vi "configureAnalogOutput.vi"(8 "error in (no error)":errorcluster, 9 "AnalogOutput":refnum<class "AnalogOutput.lvclass">, 10 "deviceName":string, 11 "AtomChipHWC in":refnum<class "AtomChipHWC.lvclass">) -> (0 "error out":errorcluster, 3 "AtomChipHWC out":refnum<class "AtomChipHWC.lvclass">)   [LabVIEW 2009, in "Hardware.lvlib" / "HWControllers.lvlib" / "AtomChipHWC.lvclass"]
doc: "Configure the analog channels of a device"
uses:
  AtomChipHWC.lvclass
  Channels/VoltOutput/AnalogOutput.lvclass
  AtomChipHWC.lvclass/AtomChipHWC.ctl
  HWController.lvclass
  Tools/Filing/FileNeologist/FileNeologist.lvclass
  Tools/Filing.lvlib
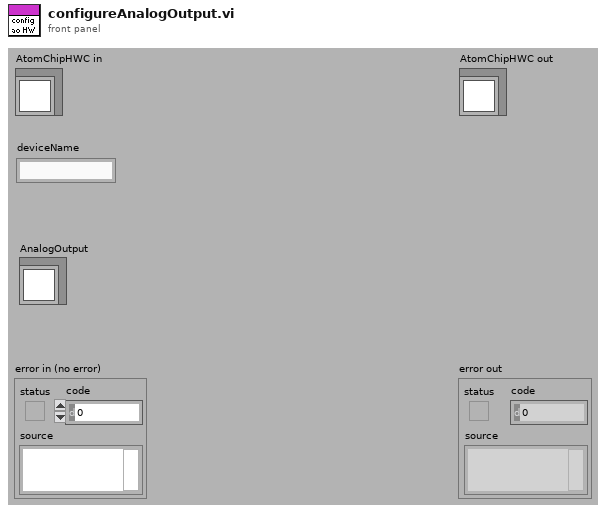
[diagram p1: front panel]
types:
  T1 = cluster{string, "Physical Channels":string, "Ranges":dbl[]}
  T2 = cluster{"Clock source":string, "Clock rate":dbl, "Start trigger line":string, "Sample Rate":dbl, "Sample No.":dbl}
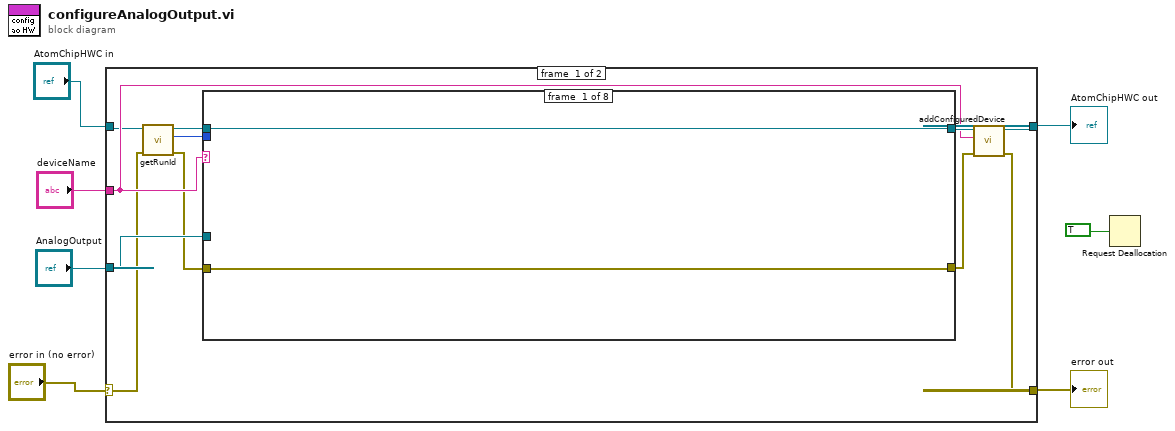
[diagram p0: block diagram]
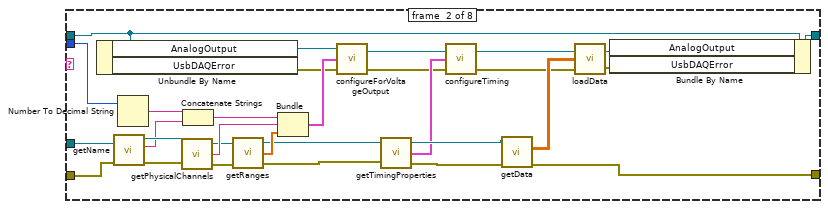
[diagram p2: hidden frame]
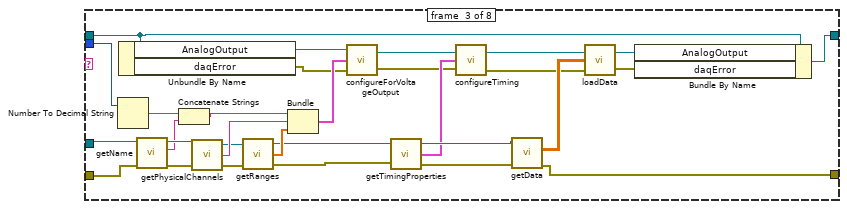
[diagram p3: hidden frame]
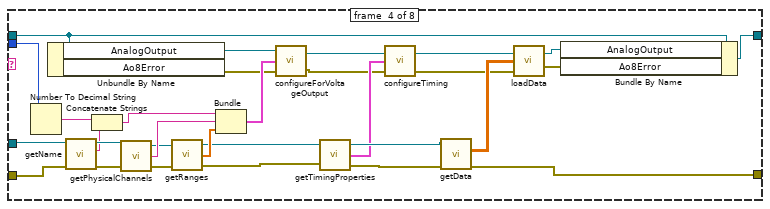
[diagram p4: hidden frame]
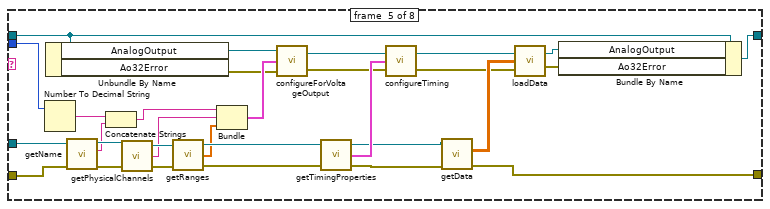
[diagram p5: hidden frame]
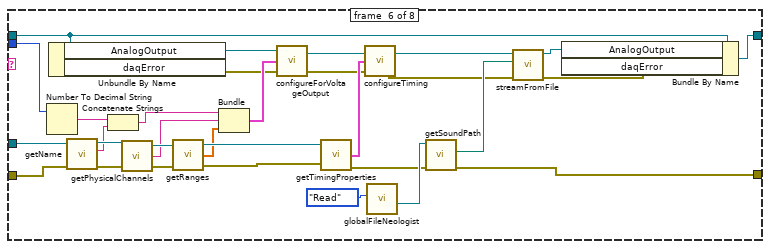
[diagram p6: hidden frame]
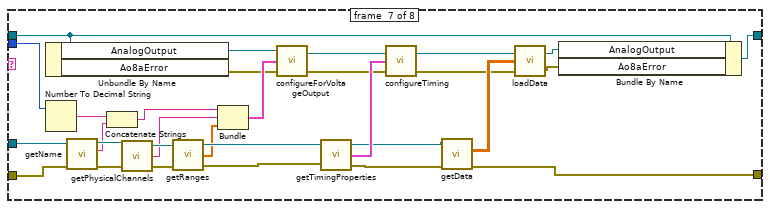
[diagram p7: hidden frame]
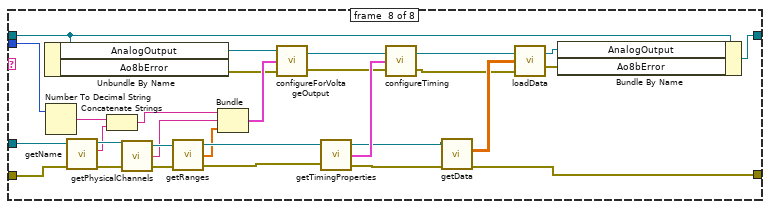
[diagram p8: hidden frame]
diagram:
  n1 = case shown="No Error" "error in (no error)" {
    selector: "error in (no error)" -> [w10 w233]
    tunnel: [w14 w233] -> w6
    tunnel: [w16 w232] -> w4
    tunnel: "AtomChipHWC in" -> [w11 w232]
    tunnel: "deviceName" -> [w13 _]
    tunnel: "AnalogOutput" -> [w18 _]
    frame #0 {
      n2 = call "getRunId.vi"("error in (no error)"=w10, "HWController in"=w11) -> ("error out"=w9:errorcluster, "Numeric"=w8:i32, "HWController out"=w12:refnum<class "AtomChipHWC.lvclass">)  [unwired: 7 in]
      n3 = case shown="\"Ao8b\"" w13 {
        tunnel: w12 -> [w20 w35 w65 w95 w140 w171 w201 w231]
        tunnel: [w20 w34 w64 w94 w139 w170 w200 w230] -> w17
        tunnel: [w19 w21 w52 w82 w113 w143 w172 w204] -> w15
        tunnel: w18 -> [_ w33 w63 w93 w132 w163 w193 w223]
        tunnel: w9 -> [w19 w32 w62 w92 w133 w164 w194 w224]
        tunnel: w8 -> [_ w28 w60 w90 w120 w155 w181 w211]
        frame #0 {
        }
        frame #1 {
          n4 = Unbundle By Name(w35) -> ("AnalogOutput"=w41:refnum<class "AnalogOutput.lvclass">, "UsbDAQError"=w24:errorcluster)
          n5 = call "getName.vi"("error in (no error)"=w32, "AnalogOutput.lvclass in"=w33) -> ("error out"=w36:errorcluster, "name"=w30:string, "AnalogOutput.lvclass out"=w38:refnum<class "AnalogOutput.lvclass">)  [unwired: 7 in]
          n6 = Number To Decimal String(number=w28) -> (decimal integer string=w31:string)  [unwired: 1 in]
          n7 = call-dynamic "getPhysicalChannels.vi"("AnalogOutput.lvclass in"=w38, "error in (no error)"=w36) -> ("AnalogOutput.lvclass out"=w39:refnum<class "AnalogOutput.lvclass">, "Physical Channels"=w42:string, "error out"=w37:errorcluster)
          n8 = Concatenate Strings(w31, w30) -> (w29:string)
          n9 = call "getRanges.vi"("AnalogOutput.lvclass in"=w39, "error in (no error)"=w37) -> ("AnalogOutput.lvclass out"=w40:refnum<class "AnalogOutput.lvclass">, "Ranges"=w43:dbl[], "error out"=w23:errorcluster)
          n10 = Bundle(w29, "Physical Channels"=w42, "Ranges"=w43) -> (w44:T1)  [unwired: 1 in]
          n11 = call-dynamic "configureForVoltageOutput.vi"("error in (no error)"=w24, "Output Properties"=w44, "AnalogOutput in"=w41) -> ("error out"=w25:errorcluster, "AnalogOutput out"=w47:refnum<class "AnalogOutput.lvclass">)
          n12 = call "getTimingProperties.vi"("AnalogOutput.lvclass in"=w40, "error in (no error)"=w23) -> ("AnalogOutput.lvclass out"=w46:refnum<class "AnalogOutput.lvclass">, "Timing"=w45:T2, "error out"=w22:errorcluster)
          n13 = call-dynamic "configureTiming.vi"("error in (no error)"=w25, "Timing"=w45, "AnalogOutput in"=w47) -> ("error out"=w26:errorcluster, "AnalogOutput out"=w48:refnum<class "AnalogOutput.lvclass">)
          n14 = call "getData.vi"("error in (no error)"=w22, "AnalogOutput.lvclass in"=w46) -> ("error out"=w21:errorcluster, "Data"=w49:dbl[][])  [unwired: 7 in, 1 out]
          n15 = call-dynamic "loadData.vi"("error in (no error)"=w26, "Data"=w49, "AnalogOutput in"=w48) -> ("error out"=w27:errorcluster, "AnalogOutput out"=w50:refnum<class "AnalogOutput.lvclass">)
          n16 = Bundle By Name(cluster=w35, "AnalogOutput"=w50, "UsbDAQError"=w27) -> (w34:refnum<class "AtomChipHWC.lvclass">)
        }
        frame #2 {
          n17 = Number To Decimal String(number=w60) -> (decimal integer string=w61:string)  [unwired: 1 in]
          n18 = Unbundle By Name(w65) -> ("AnalogOutput"=w71:refnum<class "AnalogOutput.lvclass">, "daqError"=w55:errorcluster)
          n19 = call "getName.vi"("error in (no error)"=w62, "AnalogOutput.lvclass in"=w63) -> ("error out"=w66:errorcluster, "name"=w59:string, "AnalogOutput.lvclass out"=w68:refnum<class "AnalogOutput.lvclass">)  [unwired: 7 in]
          n20 = Concatenate Strings(w61, w59) -> (w58:string)
          n21 = call-dynamic "getPhysicalChannels.vi"("AnalogOutput.lvclass in"=w68, "error in (no error)"=w66) -> ("AnalogOutput.lvclass out"=w69:refnum<class "AnalogOutput.lvclass">, "Physical Channels"=w72:string, "error out"=w67:errorcluster)
          n22 = call "getRanges.vi"("AnalogOutput.lvclass in"=w69, "error in (no error)"=w67) -> ("AnalogOutput.lvclass out"=w70:refnum<class "AnalogOutput.lvclass">, "Ranges"=w73:dbl[], "error out"=w57:errorcluster)
          n23 = Bundle(w58, "Physical Channels"=w72, "Ranges"=w73) -> (w74:T1)  [unwired: 1 in]
          n24 = call-dynamic "configureForVoltageOutput.vi"("error in (no error)"=w55, "Output Properties"=w74, "AnalogOutput in"=w71) -> ("error out"=w53:errorcluster, "AnalogOutput out"=w77:refnum<class "AnalogOutput.lvclass">)
          n25 = call "getTimingProperties.vi"("AnalogOutput.lvclass in"=w70, "error in (no error)"=w57) -> ("AnalogOutput.lvclass out"=w76:refnum<class "AnalogOutput.lvclass">, "Timing"=w75:T2, "error out"=w54:errorcluster)
          n26 = call-dynamic "configureTiming.vi"("error in (no error)"=w53, "Timing"=w75, "AnalogOutput in"=w77) -> ("error out"=w56:errorcluster, "AnalogOutput out"=w78:refnum<class "AnalogOutput.lvclass">)
          n27 = call "getData.vi"("error in (no error)"=w54, "AnalogOutput.lvclass in"=w76) -> ("error out"=w52:errorcluster, "Data"=w79:dbl[][])  [unwired: 7 in, 1 out]
          n28 = call-dynamic "loadData.vi"("error in (no error)"=w56, "Data"=w79, "AnalogOutput in"=w78) -> ("error out"=w51:errorcluster, "AnalogOutput out"=w80:refnum<class "AnalogOutput.lvclass">)
          n29 = Bundle By Name(cluster=w65, "AnalogOutput"=w80, "daqError"=w51) -> (w64:refnum<class "AtomChipHWC.lvclass">)
        }
        frame #3 {
          n30 = Number To Decimal String(number=w90) -> (decimal integer string=w91:string)  [unwired: 1 in]
          n31 = Unbundle By Name(w95) -> ("AnalogOutput"=w101:refnum<class "AnalogOutput.lvclass">, "Ao8Error"=w85:errorcluster)
          n32 = call "getName.vi"("error in (no error)"=w92, "AnalogOutput.lvclass in"=w93) -> ("error out"=w96:errorcluster, "name"=w89:string, "AnalogOutput.lvclass out"=w98:refnum<class "AnalogOutput.lvclass">)  [unwired: 7 in]
          n33 = Concatenate Strings(w91, w89) -> (w88:string)
          n34 = call-dynamic "getPhysicalChannels.vi"("AnalogOutput.lvclass in"=w98, "error in (no error)"=w96) -> ("AnalogOutput.lvclass out"=w99:refnum<class "AnalogOutput.lvclass">, "Physical Channels"=w102:string, "error out"=w97:errorcluster)
          n35 = call "getRanges.vi"("AnalogOutput.lvclass in"=w99, "error in (no error)"=w97) -> ("AnalogOutput.lvclass out"=w100:refnum<class "AnalogOutput.lvclass">, "Ranges"=w103:dbl[], "error out"=w84:errorcluster)
          n36 = Bundle(w88, "Physical Channels"=w102, "Ranges"=w103) -> (w104:T1)  [unwired: 1 in]
          n37 = call-dynamic "configureForVoltageOutput.vi"("error in (no error)"=w85, "Output Properties"=w104, "AnalogOutput in"=w101) -> ("error out"=w86:errorcluster, "AnalogOutput out"=w107:refnum<class "AnalogOutput.lvclass">)
          n38 = call "getTimingProperties.vi"("AnalogOutput.lvclass in"=w100, "error in (no error)"=w84) -> ("AnalogOutput.lvclass out"=w106:refnum<class "AnalogOutput.lvclass">, "Timing"=w105:T2, "error out"=w83:errorcluster)
          n39 = call-dynamic "configureTiming.vi"("error in (no error)"=w86, "Timing"=w105, "AnalogOutput in"=w107) -> ("error out"=w87:errorcluster, "AnalogOutput out"=w108:refnum<class "AnalogOutput.lvclass">)
          n40 = call "getData.vi"("error in (no error)"=w83, "AnalogOutput.lvclass in"=w106) -> ("error out"=w82:errorcluster, "Data"=w109:dbl[][])  [unwired: 7 in, 1 out]
          n41 = call-dynamic "loadData.vi"("error in (no error)"=w87, "Data"=w109, "AnalogOutput in"=w108) -> ("error out"=w81:errorcluster, "AnalogOutput out"=w110:refnum<class "AnalogOutput.lvclass">)
          n42 = Bundle By Name(cluster=w95, "AnalogOutput"=w110, "Ao8Error"=w81) -> (w94:refnum<class "AtomChipHWC.lvclass">)
        }
        frame #4 {
          n43 = Number To Decimal String(number=w120) -> (decimal integer string=w121:string)  [unwired: 1 in]
          n44 = Unbundle By Name(w140) -> ("AnalogOutput"=w131:refnum<class "AnalogOutput.lvclass">, "Ao32Error"=w117:errorcluster)
          n45 = call "getName.vi"("error in (no error)"=w133, "AnalogOutput.lvclass in"=w132) -> ("error out"=w138:errorcluster, "name"=w119:string, "AnalogOutput.lvclass out"=w136:refnum<class "AnalogOutput.lvclass">)  [unwired: 7 in]
          n46 = Concatenate Strings(w121, w119) -> (w118:string)
          n47 = call-dynamic "getPhysicalChannels.vi"("AnalogOutput.lvclass in"=w136, "error in (no error)"=w138) -> ("AnalogOutput.lvclass out"=w135:refnum<class "AnalogOutput.lvclass">, "Physical Channels"=w130:string, "error out"=w137:errorcluster)
          n48 = call "getRanges.vi"("AnalogOutput.lvclass in"=w135, "error in (no error)"=w137) -> ("AnalogOutput.lvclass out"=w134:refnum<class "AnalogOutput.lvclass">, "Ranges"=w129:dbl[], "error out"=w111:errorcluster)
          n49 = Bundle(w118, "Physical Channels"=w130, "Ranges"=w129) -> (w128:T1)  [unwired: 1 in]
          n50 = call-dynamic "configureForVoltageOutput.vi"("error in (no error)"=w117, "Output Properties"=w128, "AnalogOutput in"=w131) -> ("error out"=w116:errorcluster, "AnalogOutput out"=w125:refnum<class "AnalogOutput.lvclass">)
          n51 = call "getTimingProperties.vi"("AnalogOutput.lvclass in"=w134, "error in (no error)"=w111) -> ("AnalogOutput.lvclass out"=w126:refnum<class "AnalogOutput.lvclass">, "Timing"=w127:T2, "error out"=w112:errorcluster)
          n52 = call-dynamic "configureTiming.vi"("error in (no error)"=w116, "Timing"=w127, "AnalogOutput in"=w125) -> ("error out"=w115:errorcluster, "AnalogOutput out"=w124:refnum<class "AnalogOutput.lvclass">)
          n53 = call "getData.vi"("error in (no error)"=w112, "AnalogOutput.lvclass in"=w126) -> ("error out"=w113:errorcluster, "Data"=w123:dbl[][])  [unwired: 7 in, 1 out]
          n54 = call-dynamic "loadData.vi"("error in (no error)"=w115, "Data"=w123, "AnalogOutput in"=w124) -> ("error out"=w114:errorcluster, "AnalogOutput out"=w122:refnum<class "AnalogOutput.lvclass">)
          n55 = Bundle By Name(cluster=w140, "AnalogOutput"=w122, "Ao32Error"=w114) -> (w139:refnum<class "AtomChipHWC.lvclass">)
        }
        frame #5 {
          n56 = Number To Decimal String(number=w155) -> (decimal integer string=w156:string)  [unwired: 1 in]
          n57 = Unbundle By Name(w171) -> ("AnalogOutput"=w162:refnum<class "AnalogOutput.lvclass">, "daqError"=w145:errorcluster)
          n58 = call "getName.vi"("error in (no error)"=w164, "AnalogOutput.lvclass in"=w163) -> ("error out"=w169:errorcluster, "name"=w154:string, "AnalogOutput.lvclass out"=w167:refnum<class "AnalogOutput.lvclass">)  [unwired: 7 in]
          n59 = Concatenate Strings(w156, w154) -> (w153:string)
          n60 = call-dynamic "getPhysicalChannels.vi"("AnalogOutput.lvclass in"=w167, "error in (no error)"=w169) -> ("AnalogOutput.lvclass out"=w166:refnum<class "AnalogOutput.lvclass">, "Physical Channels"=w161:string, "error out"=w168:errorcluster)
          n61 = call "getRanges.vi"("AnalogOutput.lvclass in"=w166, "error in (no error)"=w168) -> ("AnalogOutput.lvclass out"=w165:refnum<class "AnalogOutput.lvclass">, "Ranges"=w160:dbl[], "error out"=w141:errorcluster)
          n62 = Bundle(w153, "Physical Channels"=w161, "Ranges"=w160) -> (w159:T1)  [unwired: 1 in]
          n63 = call-dynamic "configureForVoltageOutput.vi"("error in (no error)"=w145, "Output Properties"=w159, "AnalogOutput in"=w162) -> ("error out"=w146:errorcluster, "AnalogOutput out"=w157:refnum<class "AnalogOutput.lvclass">)
          n64 = call "getTimingProperties.vi"("AnalogOutput.lvclass in"=w165, "error in (no error)"=w141) -> ("Timing"=w158:T2, "error out"=w142:errorcluster)  [unwired: 1 out]
          n65 = call-dynamic "configureTiming.vi"("error in (no error)"=w146, "Timing"=w158, "AnalogOutput in"=w157) -> ("error out"=w147:errorcluster, "AnalogOutput out"=w152:refnum<class "AnalogOutput.lvclass">)
          n66 = call "globalFileNeologist.vi"("Action"=enum16{"Write", "Read"}."Read") -> ("FileNeologist out"=w150:refnum<class "FileNeologist.lvclass">)  [unwired: 10 in]
          n67 = call "getSoundPath.vi"("error in (no error)"=w142, "FileNeologist in"=w150) -> ("error out"=w143:errorcluster, "Path"=w148:path)  [unwired: 7 in, 1 out]
          n68 = call-dynamic "streamFromFile.vi"("error in (no error)"=w147, "Path"=w148, "AnalogOutput in"=w152) -> ("error out"=w144:errorcluster, "AnalogOutput out"=w151:refnum<class "AnalogOutput.lvclass">)  [unwired: 7 in]
          n69 = Bundle By Name(cluster=w171, "AnalogOutput"=w151, "daqError"=w144) -> (w170:refnum<class "AtomChipHWC.lvclass">)
        }
        frame #6 {
          n70 = Unbundle By Name(w201) -> ("AnalogOutput"=w192:refnum<class "AnalogOutput.lvclass">, "Ao8aError"=w176:errorcluster)
          n71 = Number To Decimal String(number=w181) -> (decimal integer string=w182:string)  [unwired: 1 in]
          n72 = call "getName.vi"("error in (no error)"=w194, "AnalogOutput.lvclass in"=w193) -> ("error out"=w199:errorcluster, "name"=w180:string, "AnalogOutput.lvclass out"=w197:refnum<class "AnalogOutput.lvclass">)  [unwired: 7 in]
          n73 = Concatenate Strings(w182, w180) -> (w179:string)
          n74 = call-dynamic "getPhysicalChannels.vi"("AnalogOutput.lvclass in"=w197, "error in (no error)"=w199) -> ("AnalogOutput.lvclass out"=w196:refnum<class "AnalogOutput.lvclass">, "Physical Channels"=w191:string, "error out"=w198:errorcluster)
          n75 = call "getRanges.vi"("AnalogOutput.lvclass in"=w196, "error in (no error)"=w198) -> ("AnalogOutput.lvclass out"=w195:refnum<class "AnalogOutput.lvclass">, "Ranges"=w190:dbl[], "error out"=w173:errorcluster)
          n76 = Bundle(w179, "Physical Channels"=w191, "Ranges"=w190) -> (w189:T1)  [unwired: 1 in]
          n77 = call-dynamic "configureForVoltageOutput.vi"("error in (no error)"=w176, "Output Properties"=w189, "AnalogOutput in"=w192) -> ("error out"=w177:errorcluster, "AnalogOutput out"=w186:refnum<class "AnalogOutput.lvclass">)
          n78 = call "getTimingProperties.vi"("AnalogOutput.lvclass in"=w195, "error in (no error)"=w173) -> ("AnalogOutput.lvclass out"=w187:refnum<class "AnalogOutput.lvclass">, "Timing"=w188:T2, "error out"=w174:errorcluster)
          n79 = call-dynamic "configureTiming.vi"("error in (no error)"=w177, "Timing"=w188, "AnalogOutput in"=w186) -> ("error out"=w178:errorcluster, "AnalogOutput out"=w185:refnum<class "AnalogOutput.lvclass">)
          n80 = call "getData.vi"("error in (no error)"=w174, "AnalogOutput.lvclass in"=w187) -> ("error out"=w172:errorcluster, "Data"=w184:dbl[][])  [unwired: 7 in, 1 out]
          n81 = call-dynamic "loadData.vi"("error in (no error)"=w178, "Data"=w184, "AnalogOutput in"=w185) -> ("error out"=w175:errorcluster, "AnalogOutput out"=w183:refnum<class "AnalogOutput.lvclass">)
          n82 = Bundle By Name(cluster=w201, "AnalogOutput"=w183, "Ao8aError"=w175) -> (w200:refnum<class "AtomChipHWC.lvclass">)
        }
        frame #7 {
          n83 = Unbundle By Name(w231) -> ("AnalogOutput"=w222:refnum<class "AnalogOutput.lvclass">, "Ao8bError"=w208:errorcluster)
          n84 = Number To Decimal String(number=w211) -> (decimal integer string=w212:string)  [unwired: 1 in]
          n85 = call "getName.vi"("error in (no error)"=w224, "AnalogOutput.lvclass in"=w223) -> ("error out"=w229:errorcluster, "name"=w210:string, "AnalogOutput.lvclass out"=w227:refnum<class "AnalogOutput.lvclass">)  [unwired: 7 in]
          n86 = Concatenate Strings(w212, w210) -> (w209:string)
          n87 = call-dynamic "getPhysicalChannels.vi"("AnalogOutput.lvclass in"=w227, "error in (no error)"=w229) -> ("AnalogOutput.lvclass out"=w226:refnum<class "AnalogOutput.lvclass">, "Physical Channels"=w221:string, "error out"=w228:errorcluster)
          n88 = call "getRanges.vi"("AnalogOutput.lvclass in"=w226, "error in (no error)"=w228) -> ("AnalogOutput.lvclass out"=w225:refnum<class "AnalogOutput.lvclass">, "Ranges"=w220:dbl[], "error out"=w202:errorcluster)
          n89 = Bundle(w209, "Physical Channels"=w221, "Ranges"=w220) -> (w219:T1)  [unwired: 1 in]
          n90 = call-dynamic "configureForVoltageOutput.vi"("error in (no error)"=w208, "Output Properties"=w219, "AnalogOutput in"=w222) -> ("error out"=w207:errorcluster, "AnalogOutput out"=w216:refnum<class "AnalogOutput.lvclass">)
          n91 = call "getTimingProperties.vi"("AnalogOutput.lvclass in"=w225, "error in (no error)"=w202) -> ("AnalogOutput.lvclass out"=w217:refnum<class "AnalogOutput.lvclass">, "Timing"=w218:T2, "error out"=w203:errorcluster)
          n92 = call-dynamic "configureTiming.vi"("error in (no error)"=w207, "Timing"=w218, "AnalogOutput in"=w216) -> ("error out"=w206:errorcluster, "AnalogOutput out"=w215:refnum<class "AnalogOutput.lvclass">)
          n93 = call "getData.vi"("error in (no error)"=w203, "AnalogOutput.lvclass in"=w217) -> ("error out"=w204:errorcluster, "Data"=w214:dbl[][])  [unwired: 7 in, 1 out]
          n94 = call-dynamic "loadData.vi"("error in (no error)"=w206, "Data"=w214, "AnalogOutput in"=w215) -> ("error out"=w205:errorcluster, "AnalogOutput out"=w213:refnum<class "AnalogOutput.lvclass">)
          n95 = Bundle By Name(cluster=w231, "AnalogOutput"=w213, "Ao8bError"=w205) -> (w230:refnum<class "AtomChipHWC.lvclass">)
        }
      }
      n96 = call "addConfiguredDevice.vi"("error in (no error)"=w15, "deviceName"=w13, "HWController in"=w17) -> ("error out"=w14:errorcluster, "HWController out"=w16:refnum<class "AtomChipHWC.lvclass">)  [unwired: 7 in]
    }
    frame #1 {
    }
  }
  "error out" <- w6
  "AtomChipHWC out" <- w4
  n97 = Request Deallocation(TRUE) -> ()
